vi "Insert Subroutine.vi"(8 "error in (no error)":errorcluster, 10 "Insert Subroutine":T1, 11 "Test Executive Builder Model in":refnum<class "Test Executive Builder Model.lvclass">) -> (0 "error out":errorcluster, 3 "Test Executive Builder Model out":refnum<class "Test Executive Builder Model.lvclass">, 5 "Unique ID out":string)   [LabVIEW 2017, in "Test Executive Builder Model.lvclass"]
uses:
  Test Executive Builder Model.lvclass
  <vilib>/gpm_packages/@cs/test-executive/Source/Test Executive/TestExecutive Ref/TestExecutive Ref.lvclass
  Test Executive Builder Model Messages/Redraw Tree Msg/Redraw Tree Msg.lvclass
  <vilib>/ActorFramework/Actor/Actor.lvclass
  C:/Program Files (x86)/National Instruments/LabVIEW 2017/vi.lib/ActorFramework/Actor/Actor.lvclass
  Application Dependencies/Insert Subroutine.ctl
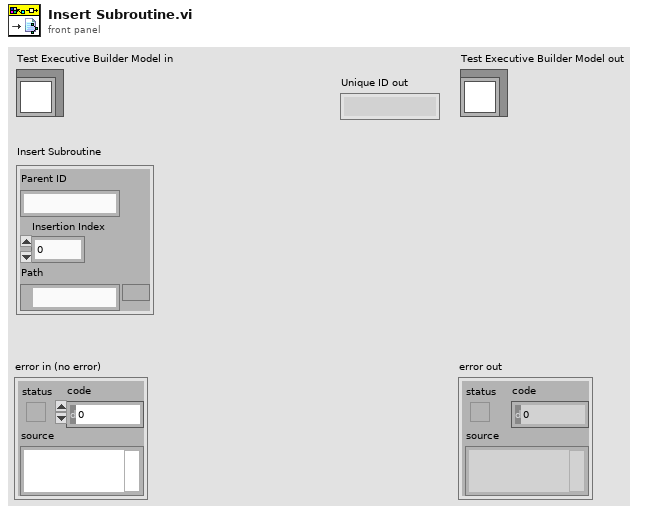
[diagram p1: front panel]
types:
  T1 = typedef "Insert Subroutine.ctl" = cluster{"Parent ID":string, "Insertion Index":i32, "Path":path}
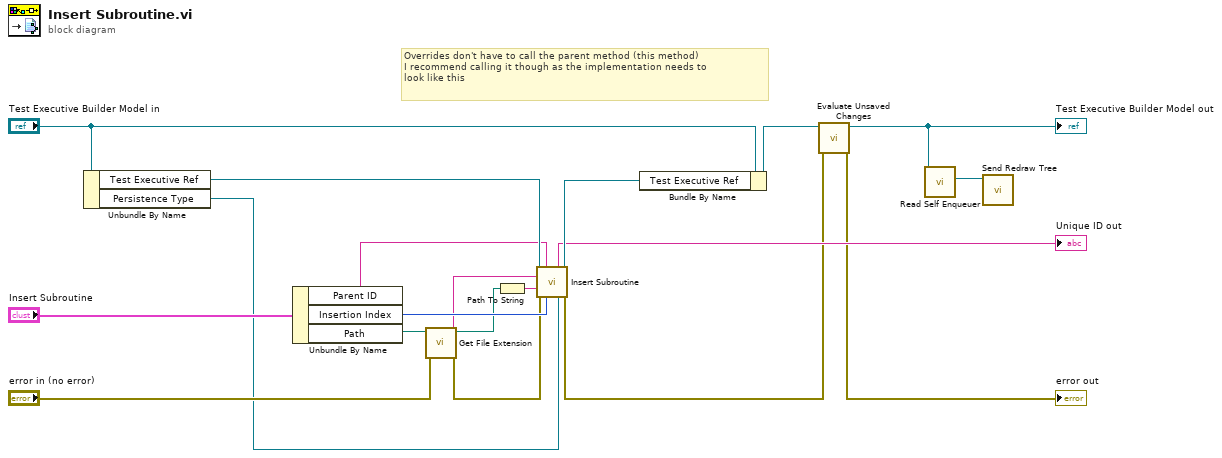
[diagram p0: block diagram]
diagram:
  # "Overrides don't have to call the parent method (this method)\nI recommend calling it though as the implementation needs to\nlook like this"
  n1 = Unbundle By Name("Test Executive Builder Model in") -> ("Test Executive Ref"=w18:refnum<data-value>, "Persistence Type"=w1:refnum<class "IPersist.lvclass">)
  n2 = Unbundle By Name("Insert Subroutine") -> ("Parent ID"=w15:string, "Insertion Index"=w14:i32, "Path"=w13:path)
  n3 = call <vilib>:"Get File Extension.vi"("error in (no error)"="error in (no error)", "file"=w13) -> ("error out"=w9:errorcluster, "filename without extension"=w12:string, "dup file"=w11:path)  [unwired: 5 in, 2 out]
  n4 = Path To String(path=w11) -> (string=w6:string)
  n5 = call <vilib>:"Insert Subroutine.vi"("Test Executive Ref"=w18, "Parent ID"=w15, "Name"=w12, "Subroutine Path"=w6, "error in (no error)"=w9, "Insertion Index"=w14, "Persistence"=w1) -> ("Unique ID out"=→"Unique ID out":string, "Test Executive Ref out"=w16:refnum<data-value>, "error out"=w3:errorcluster)  [unwired: 5 in, 1 out]
  n6 = Bundle By Name(cluster="Test Executive Builder Model in", "Test Executive Ref"=w16) -> (w5:refnum<class "Test Executive Builder Model.lvclass">)
  n7 = call-dynamic "Evaluate Unsaved Changes.vi"("error in (no error)"=w3, "Test Executive Builder Model in"=w5) -> ("error out"=→"error out":errorcluster, "Test Executive Builder Model out"=w4:refnum<class "Test Executive Builder Model.lvclass">)  [unwired: 8 in]
  "Test Executive Builder Model out" <- w4
  n8 = call <vilib>:"Read Self Enqueuer.vi"("Actor"=w4) -> ("Self Enqueuer"=w7:refnum<class "Message Enqueuer.lvclass">)  [unwired: 10 in]
  n9 = call "Send Redraw Tree.vi"("Message Enqueuer"=w7) -> ()  [unwired: 9 in, 2 out]
